vi "subAxopatch_GenSealTestWave_New.vi"(8 "Error in (no error)":errorcluster, 11 "Pipet tuning parameters":T2={"Amplitude (mV)"=5.0, "Number of repeats"=20, "Sampling rate (Hz)"=20000.0, "Wave Freq. (Hz)"=10.0}) -> (0 "Error out":errorcluster, 3 "Patch seal test wavefrom":waveform(dbl)(graph)={"t0"=timestamp(0 s since 1904-01-01), "dt"=5e-05, "Y"=array[40000 elements]}, 5 "Seal test DAQ params":T1={"samples"=40000, "Duration (sec)"=2.0, "Downsampling factor"=2000.0})   [LabVIEW 2015]
uses:
  <vilib>/Analysis/Matrix/Numeric/Conversions/Matrix To Array - RM.vi
  <vilib>/Analysis/Matrix/NI_Matrix.lvlib
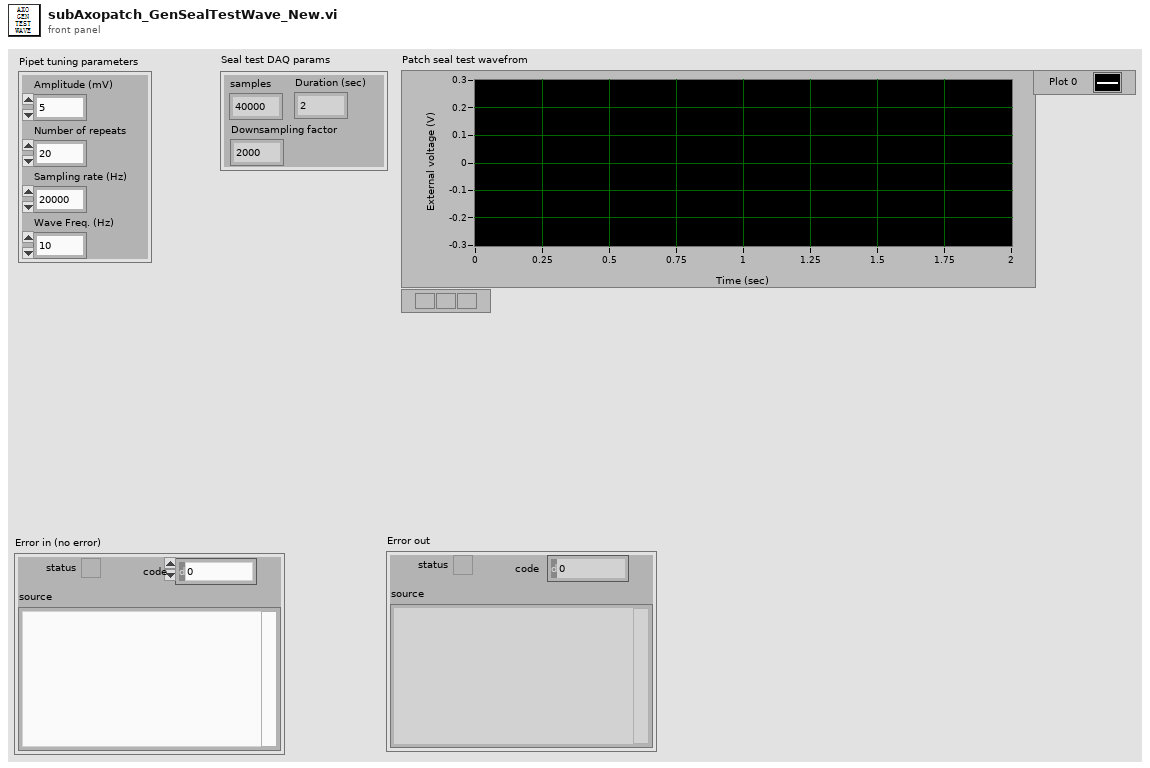
[diagram p1: front panel]
types:
  T1 = cluster{"samples":i32, "Duration (sec)":dbl, "Downsampling factor":dbl}
  T2 = cluster{"Amplitude (mV)":dbl, "Number of repeats":i32, "Sampling rate (Hz)":dbl, "Wave Freq. (Hz)":dbl}
  T3 = typedef "NI_Matrix.lvlib/RealMatrix.ctl" = dbl[][]
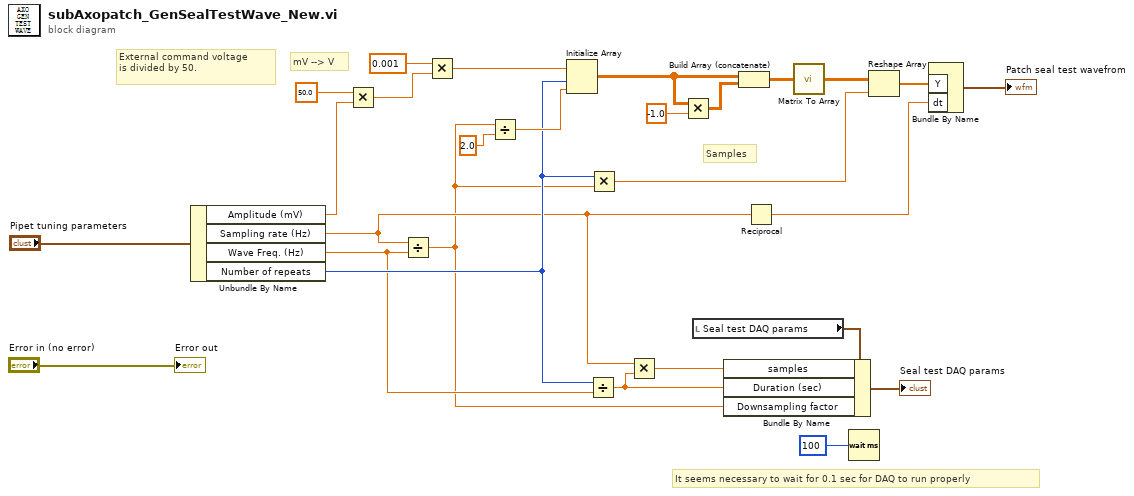
[diagram p0: block diagram]
diagram:
  # "Samples"
  # "It seems necessary to wait for 0.1 sec for DAQ to run properly"
  # "mV --> V"
  # "External command voltage\nis divided by 50."
  n1 = Unbundle By Name("Pipet tuning parameters") -> ("Amplitude (mV)"=w27:dbl, "Sampling rate (Hz)"=w3:dbl, "Wave Freq. (Hz)"=w5:dbl, "Number of repeats"=w6:i32)
  n2 = Multiply(x=50.0, y=w27) -> (x*y=w23:dbl)
  n3 = Divide(x=w3, y=w5) -> (x/y=w1:dbl)
  n4 = Multiply(x=0.001, y=w23) -> (x*y=w16:dbl)
  n5 = Divide(x=w1, y=2.0 ("x")) -> (x/y=w17:dbl)
  n6 = Initialize Array(w16, w6, w17) -> (w10:dbl[][])
  n7 = Divide(x=w6, y=w5) -> (x/y=w4:dbl)
  n8 = Multiply(x=w6, y=w1) -> (x*y=w8:dbl)
  n9 = Multiply(x=w3, y=w4) -> (x*y=w2:dbl)
  n10 = Multiply(x=w10, y=-1.0) -> (x*y=w14:dbl[][])
  n11 = local read "Seal test DAQ params"() -> (w19:T1)
  n12 = Bundle By Name(cluster=w19, "samples"=w2, "Duration (sec)"=w4, "Downsampling factor"=w1) -> (→"Seal test DAQ params":T1)
  n13 = Build Array (concatenate)(w10, w14) -> (w11:T3)
  n14 = Reciprocal(x=w3) -> (1/x=w9:dbl)
  n15 = call-poly <vilib>:"Matrix To Array.vi"("Real Matrix"=w11) -> ("Real 2D Array"=w12:dbl[][])
  n16 = Wait (ms)(milliseconds to wait=u32 100) -> ()  [unwired: 1 out]
  n17 = Reshape Array(w12, w8) -> (w13:dbl[])
  n18 = Bundle By Name("Y"=w13, "dt"=w9) -> (→"Patch seal test wavefrom":waveform(dbl))  [unwired: 1 in]
  "Error out" <- "Error in (no error)"
